vi "robot_dis.vi"() -> ()   [LabVIEW 2014]
uses:
  <vilib>/robotics/Controls/2D Rangefinder/NI_Robotics_2D Rangefinder.xctl
  <vilib>/Utility/error.llb/DialogType.ctl
  <vilib>/picture/3D Picture Control/Object/Create Object (drawable).vi
  <vilib>/picture/3D Picture Control/Object/Add Object (reference).vi
  <vilib>/picture/3D Picture Control/NI_3D Picture Control.lvlib
panel:
  out "StartChannelRecord":bool
  out "StartChannelRecord 3":bool
  out "StartChannelRecord 2":bool
  in  "AUTO":bool
  out "三维图片":refnum<vi>(3d-picture)
  out "当前方向":u8
  in  "云台枚举":enum16{"停", "上", "下", "左", "右"}(ring)
  in  "Color 2":T1={"Red"=1.0, "Green"=0.0, "Blue"=0.0, "Alpha"=1.0} caption="颜色"
  in  "Color":T1={"Red"=1.0, "Green"=0.0, "Blue"=0.0, "Alpha"=1.0} caption="颜色"
  out "小车启动":bool
  out "Lidar_two":i32
  in  "选项卡控件":T2
  out "当前速度":u16
  out "当前拉力":u16
  out "前距离(cm)":u16(slide) scale=0.0..10000.0
  out "后距离(cm)":u16(slide) scale=0.0..10000.0
  out "PITCH":i32
  out "BANK":i32
  out "HEANDING":i32
  out "当前方向":enum16{"停", "上", "下", "左", "右"}(ring)
  in  "开始后录像":bool
  in  "开始主录像":bool
  in  "开始前录像":bool
  out "前距离警告":bool
  out "后距离警告":bool
  in  "车 上":bool
  in  "车下":bool
  in  "车左":bool
  in  "加速":bool
  in  "减速":bool
  in  "车右":bool
  in  "焦距缩进":bool
  in  "焦距拉远":bool
  in  "焦点远":bool
  in  "焦点近":bool
  in  "云台右":bool
  in  "云台上":bool
  in  "云台左":bool
  in  "云台下":bool
  in  "切换备用电池":bool
  in  "绕线盘停止":bool
  in  "绕线盘反转":bool
  in  "绕线盘正转":bool
  in  "绕线转速":u16(slide) step=1 scale=500.0..10000.0
  in  "LED4":u8(slide) step=1 scale=0.0..100.0
  in  "LED3":u8(slide) step=1 scale=0.0..100.0
  in  "LED2":u8(slide) step=1 scale=0.0..100.0
  in  "LED1":u8(slide) step=1 scale=0.0..100.0
  in  "拉力上限":u16(slide) scale=0.0..2000.0
  in  "拉力下限":u16(slide) scale=0.0..2000.0
  in  "退出绕线盘模式":bool
  out "控制器":dbl(slide) scale=10.0..13.0
  out "绕线盘":dbl(slide) scale=10.0..13.0 scale format="%.3f"
  out "布尔 3":bool=TRUE
  out "StartChannelRealPlay":bool
  in  "Lidar_data":cluster{"数组":dbl[], "数组 2":dbl[][]}
  out "Rangefinder Indicator":cluster{"angle":dbl[], "distance":dbl[][]}(xcontrol)
  out "扫描质量":u8
  out "Lidar_size":u16
  in  "distance":dbl[](array[numeric])
  in  "angle":dbl[](array[numeric])
  out "数值 2":u8 format="%x"
  out "x或y?":u8 format="%x"
  out "x = y?":bool
  out "无符号字节数组 2":u8[](array[numeric])
  out "动力":dbl(slide) scale=10.0..13.0
  in  "控制电量":dbl(slide) scale=0.0..100.0
  in  "主摄像头":refnum<k7>(container)
  in  "后摄像头":refnum<k7>(container)
  out "Login 2":i32
  out "前摄像头":bool
  out "后摄像头":bool
  out "Login":i32
  in  "前摄像头":refnum<k7>(container)
  in  "缩放":dbl(knob)=2.2771854734286614 scale=0.0..10.0
  in  "方向枚举":enum16{"停", "上", "下", "左", "右"}(ring)
  out "和":u8
  out "小车锁定":u8
  out "数据传输":bool
  in  "数据输入":string
  in  "QUIT":bool
  in  "WRITE":bool
  # "TETRAELC--机器人测试平台V0.1"
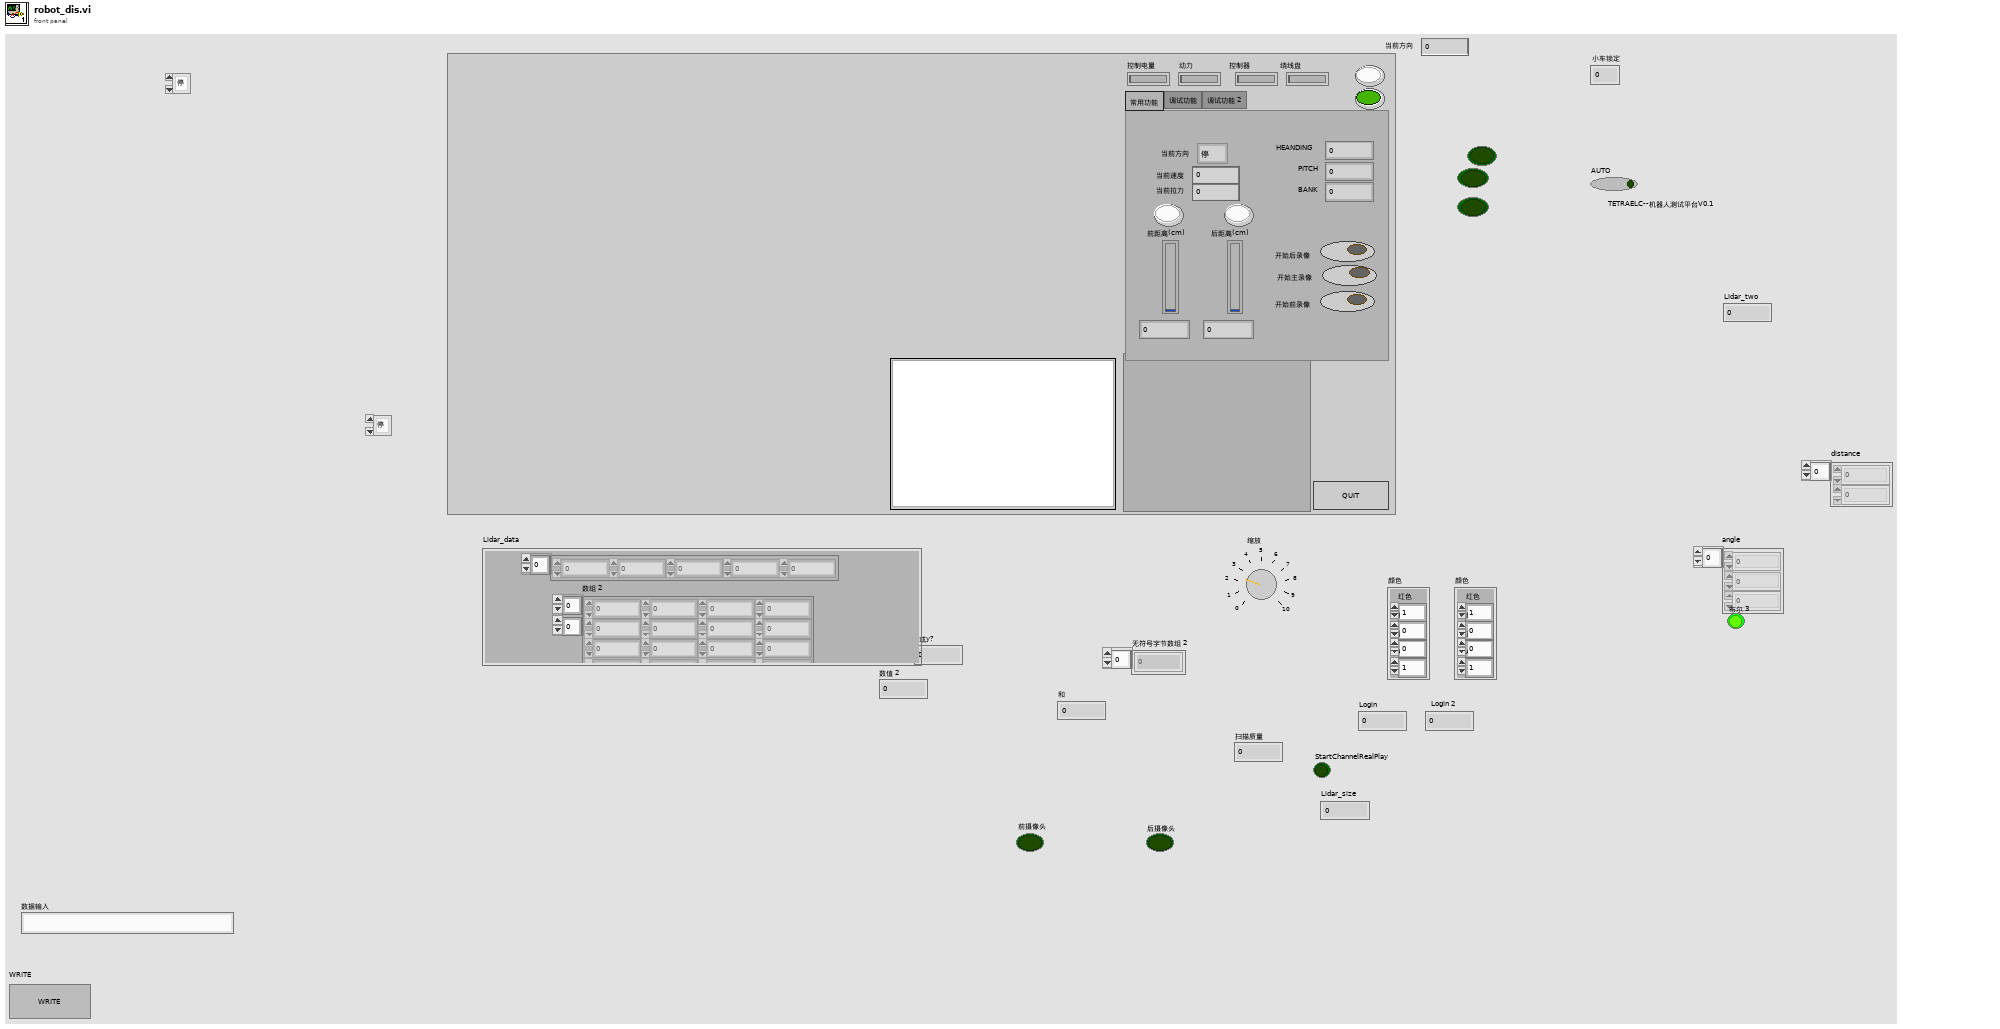
[diagram p1: front panel]
types:
  T1 = cluster{"Red":sgl, "Green":sgl, "Blue":sgl, "Alpha":sgl}
  T2 = typedef "选项卡.ctl" = enum32{"常用功能", "调试功能", "调试功能 2"}
  T3 = typedef "DialogType.ctl" = u16
  T4 = cluster{"Car_lock":u8, "当前方向":u8, "当前速度\n":u16, "当前拉力":u16}
  T5 = cluster{"PITCH":i32, "BANK":i32, "HEANDING":i32, "X":i32, "Y":i32, "Z":i32}
  T6 = cluster{"quality":u8, "angle":u16, "distance\n":u16}
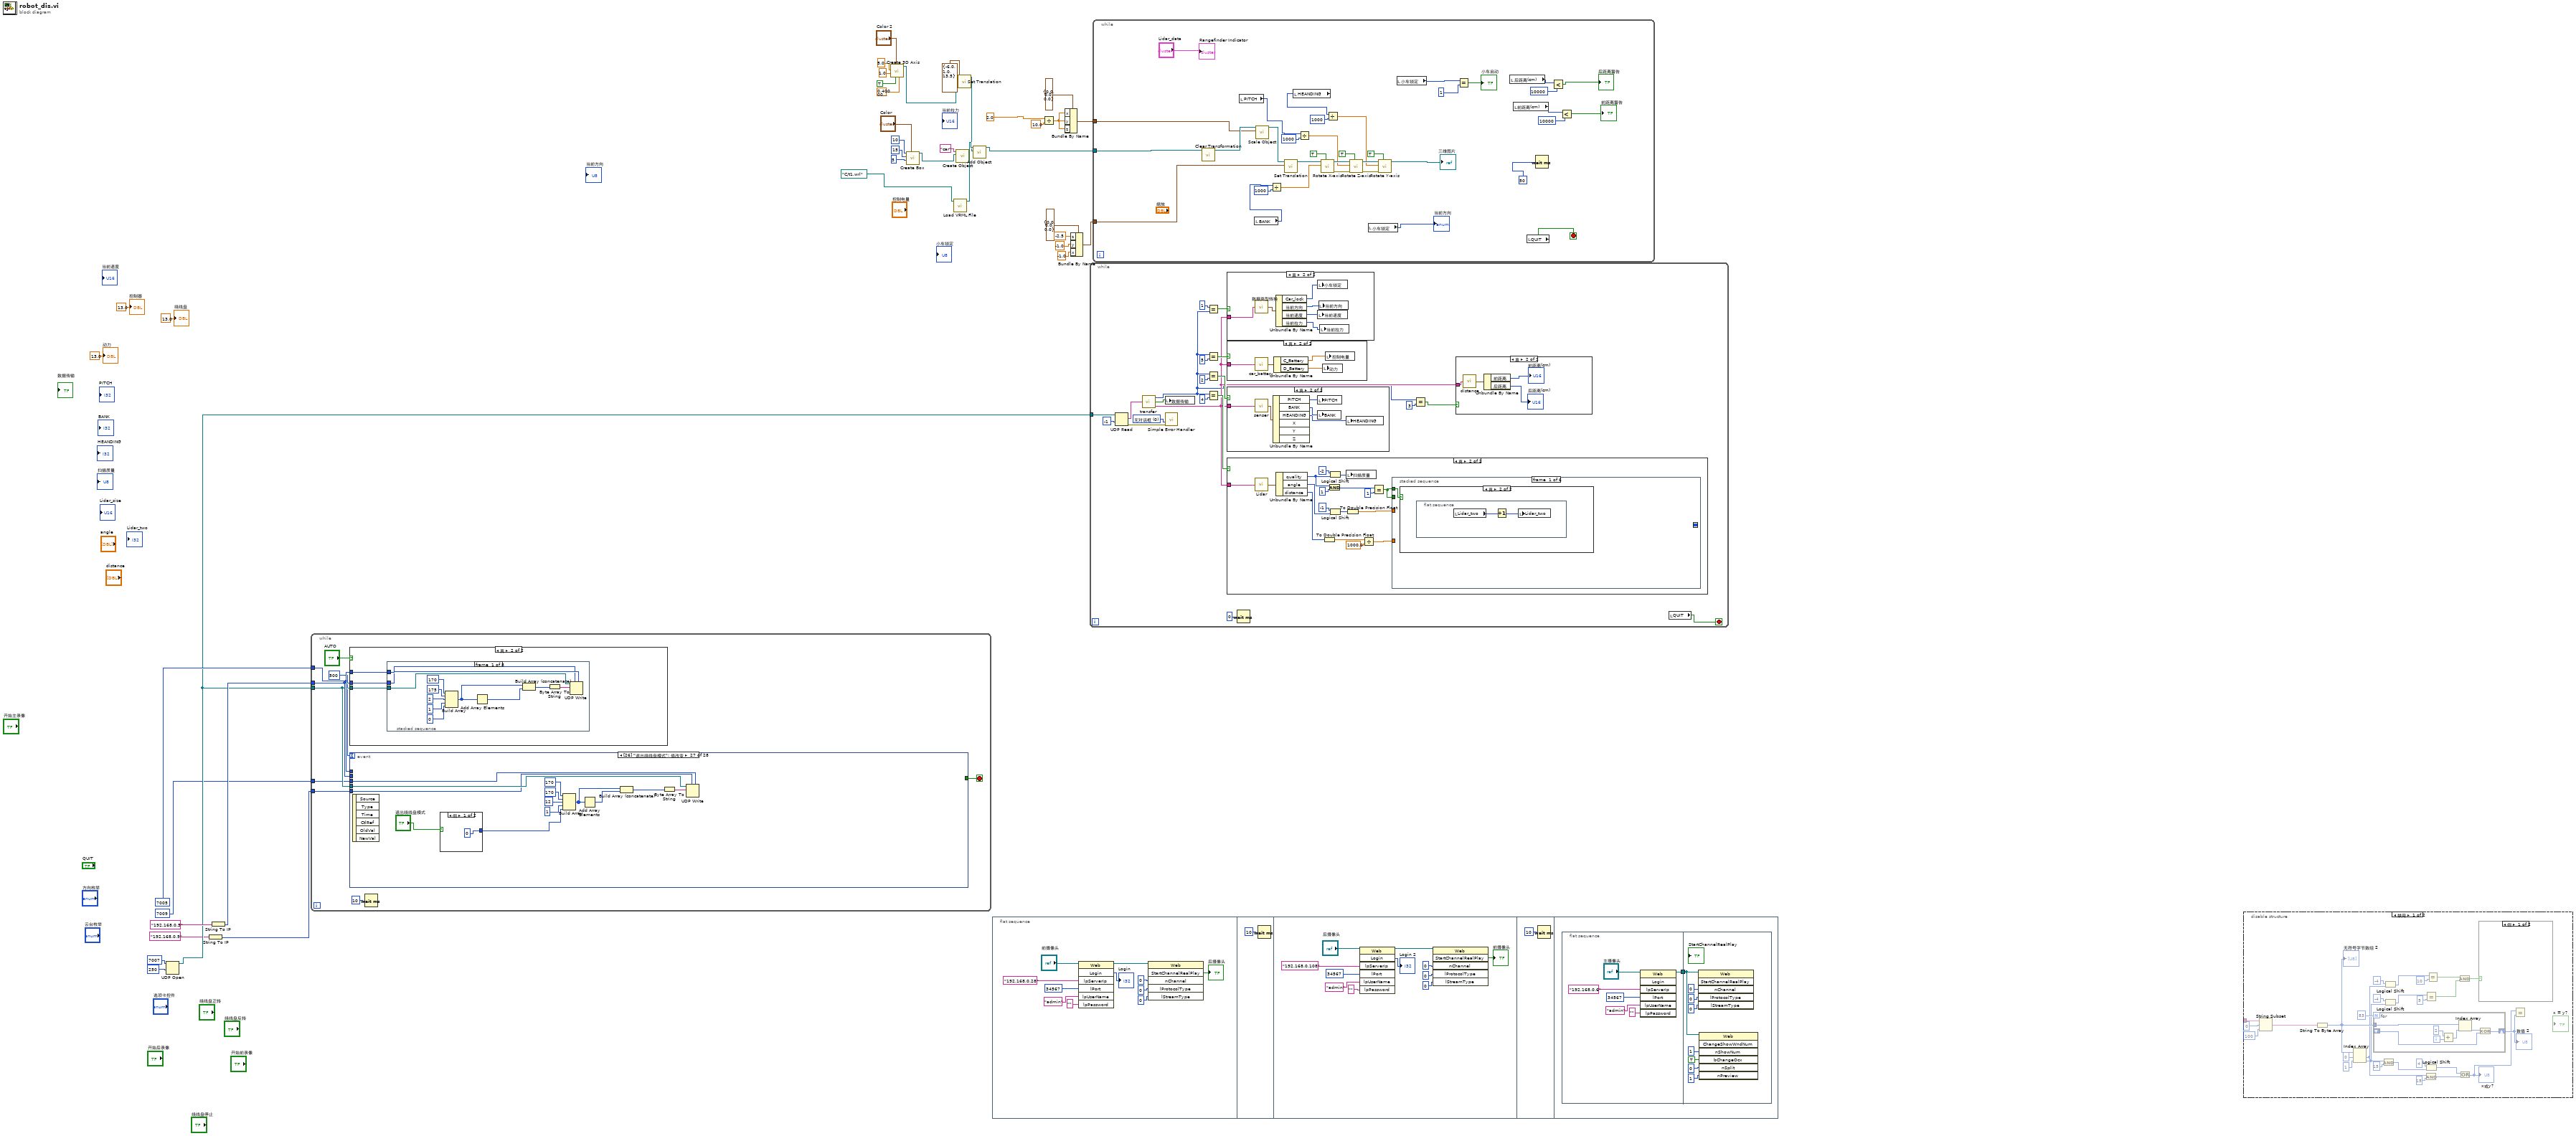
[diagram p0: block diagram]
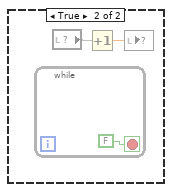
[diagram p2: hidden frame]
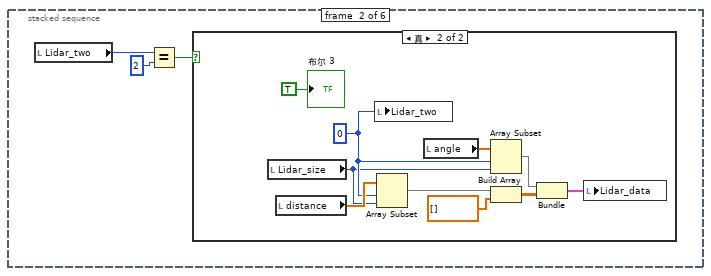
[diagram p7: hidden frame]
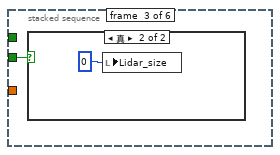
[diagram p9: hidden frame]
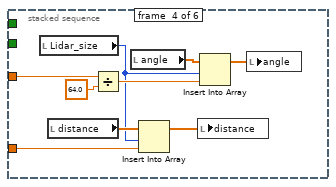
[diagram p11: hidden frame]
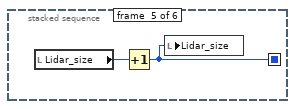
[diagram p12: hidden frame]
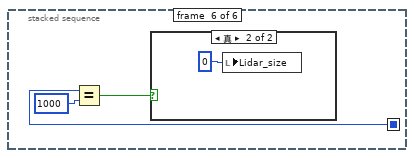
[diagram p13: hidden frame]
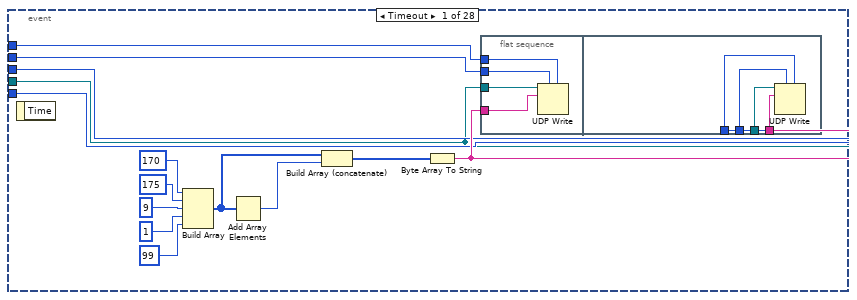
[diagram p18: hidden frame]
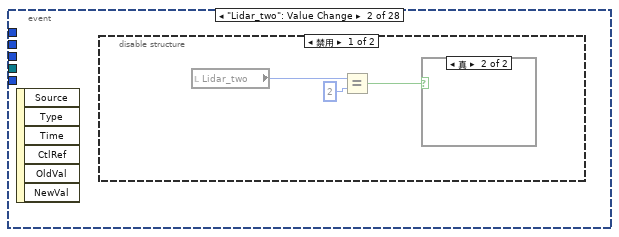
[diagram p19: hidden frame]
diagram:
  n1 = UDP Open(9:250 ("超时毫秒(25000)"), 11:u16 7007 ("本地端口")) -> (port=w26:refnum<k16>)  [unwired: 3 in, 2 out]
  n2 = String To IP(1:"192.168.0.9" ("目标主机")) -> (0:w22:u32)
  n3 = String To IP(1:"192.168.0.5" ("目标主机")) -> (0:w37:u32)
  n4 = while {
    tunnel: w26 -> [w46]
    tunnel: w37 -> [w47]
    tunnel: u16 7005 ("目标端口") -> [w48]
    tunnel: w22 -> [w41]
    tunnel: u16 7009 ("目标端口") -> [w40]
    stop <- w42 stop-if-true
    n5 = case shown="真" "AUTO" {
      tunnel: w48 -> [_ w474]
      tunnel: w47 -> [_ w473]
      tunnel: w46 -> [_ w472]
      frame False {
      }
      frame True {
        n6 = stacked-sequence {
          tunnel: w474 -> [w477 _ w488 _ w502 _ w515 _]
          tunnel: w473 -> [w476 _ w489 _ w503 _ w516 _]
          tunnel: w472 -> [w475 _ w490 _ w504 _ w514 _]
          frame #0 {
            n7 = Build Array(u8 170 ("元素"), u8 175 ("元素"), u8 2 ("元素"), u8 1 ("元素"), u8 0 ("元素")) -> (w481:u8[])
            n8 = Add Array Elements(numeric array=w481) -> (sum=w480:u8)
            n9 = Build Array (concatenate)(w481, w480) -> (w479:u8[])
            n10 = Byte Array To String(unsigned byte array=w479) -> (string=w486:string)
            n11 = UDP Write(address=w476, port or service name=w477, connection ID=w475, data in=w486) -> ()  [unwired: 2 in, 2 out]
          }
          frame #1 {
            n12 = Wait (ms)(milliseconds to wait=u32 3000 ("等待时间（毫秒）")) -> ()  [unwired: 1 out]
          }
          frame #2 {
            n13 = Build Array(u8 170 ("元素"), u8 175 ("元素"), u8 2 ("元素"), u8 1 ("元素"), u8 8 ("元素")) -> (w494:u8[])
            n14 = Add Array Elements(numeric array=w494) -> (sum=w493:u8)
            n15 = Build Array (concatenate)(w494, w493) -> (w492:u8[])
            n16 = Byte Array To String(unsigned byte array=w492) -> (string=w499:string)
            n17 = UDP Write(address=w489, port or service name=w488, connection ID=w490, data in=w499) -> ()  [unwired: 2 in, 2 out]
          }
          frame #3 {
            n18 = Wait (ms)(milliseconds to wait=u32 1000 ("等待时间（毫秒）")) -> ()  [unwired: 1 out]
          }
          frame #4 {
            n19 = Build Array(u8 170 ("元素"), u8 175 ("元素"), u8 2 ("元素"), u8 1 ("元素"), u8 1 ("元素")) -> (w508:u8[])
            n20 = Add Array Elements(numeric array=w508) -> (sum=w507:u8)
            n21 = Build Array (concatenate)(w508, w507) -> (w506:u8[])
            n22 = Byte Array To String(unsigned byte array=w506) -> (string=w512:string)
            n23 = UDP Write(address=w503, port or service name=w502, connection ID=w504, data in=w512) -> ()  [unwired: 2 in, 2 out]
          }
          frame #5 {
            n24 = Wait (ms)(milliseconds to wait=u32 3000 ("等待时间（毫秒）")) -> ()  [unwired: 1 out]
          }
          frame #6 {
            n25 = Build Array(u8 170 ("元素"), u8 175 ("元素"), u8 2 ("元素"), u8 1 ("元素"), u8 8 ("元素")) -> (w520:u8[])
            n26 = Add Array Elements(numeric array=w520) -> (sum=w519:u8)
            n27 = Build Array (concatenate)(w520, w519) -> (w518:u8[])
            n28 = Byte Array To String(unsigned byte array=w518) -> (string=w525:string)
            n29 = UDP Write(address=w516, port or service name=w515, connection ID=w514, data in=w525) -> ()  [unwired: 2 in, 2 out]
          }
          frame #7 {
            n30 = Wait (ms)(milliseconds to wait=u32 1000 ("等待时间（毫秒）")) -> ()  [unwired: 1 out]
          }
        }
      }
    }
    n31 = event shown="[26] \"退出绕线盘模式\": 值改变" {
      selector: _ -> [_ _ _ _ _ _ _ _ _ _ _ _ _ _ _ _ _ _ _ _ _ _ _ _ _ _ _ _]
      dyn-events: _ -> [_ _ _ _ _ _ _ _ _ _ _ _ _ _ _ _ _ _ _ _ _ _ _ _ _ _ _ _]
      timeout: 500 -> [_ _ _ _ _ _ _ _ _ _ _ _ _ _ _ _ _ _ _ _ _ _ _ _ _ _ _ _]
      tunnel: w46 -> [w49 _ _ _ _ w114 w131 _ _ _ _ w191 w205 w226 w250 w270 w300 w309 w331 w353 w377 w389 w399 w416 w428 w430 w440 w455]
      tunnel: w47 -> [w54 _ _ _ _ w115 w132 _ _ _ _ w192 w206 w227 w249 w271 _ w310 w332 w354 _ _ _ _ w427 _ _ w453]
      tunnel: w48 -> [w55 _ _ _ _ w116 w133 _ _ _ _ w193 w207 w228 w248 w272 _ w311 w333 w355 _ _ _ _ w426 _ _ w454]
      tunnel: [_ _ _ _ _ _ _ _ _ _ _ _ _ _ _ _ _ _ _ _ _ _ _ _ _ w429 _ _] -> w42
      tunnel: w41 -> [w51 _ _ _ _ _ _ _ _ _ _ _ _ _ _ _ w298 _ _ _ w376 w388 w401 w411 _ _ w439 _]
      tunnel: w40 -> [w50 _ _ _ _ _ _ _ _ _ _ _ _ _ _ _ w299 _ _ _ w375 w387 w400 w412 _ _ w441 _]
      event Timeout {
        n32 = event-data() -> ()  [unwired: 1 in, 1 out]
        n33 = Build Array(u8 170 ("元素"), u8 175 ("元素"), u8 9 ("元素"), u8 1 ("元素"), u8 99 ("元素")) -> (w58:u8[])
        n34 = Add Array Elements(numeric array=w58) -> (sum=w57:u8)
        n35 = Build Array (concatenate)(w58, w57) -> (w56:u8[])
        n36 = Byte Array To String(unsigned byte array=w56) -> (string=w52:string)
        n37 = flat-sequence {
          tunnel: w55 -> [w66]
          tunnel: w54 -> [w65]
          tunnel: w52 -> [w64]
          tunnel: w49 -> [w63]
          tunnel: w52 -> [w70]
          tunnel: w51 -> [w69]
          tunnel: w50 -> [w68]
          tunnel: w49 -> [w67]
          frame #0 {
            n38 = UDP Write(address=w65, port or service name=w66, connection ID=w63, data in=w64) -> ()  [unwired: 2 in, 2 out]
          }
          frame #1 {
            n39 = UDP Write(address=w69, port or service name=w68, connection ID=w67, data in=w70) -> ()  [unwired: 2 in, 2 out]
          }
        }
      }
      event "Lidar_two": Value Change {
        n40 = event-data() -> ()  [unwired: 1 in, 6 out]
        n41 = disable-structure shown="禁用" {
          frame Disabled {
            n42 = local read "Lidar_two"() -> (w73:i32)
            n43 = Equal?(x=w73, y=2) -> (x = y?=w71:bool)
            n44 = case shown="真" w71 {
              frame False {
              }
              frame True {
              }
            }
          }
          frame Enabled {
          }
        }
      }
      event "开始主录像": Value Change {
        n45 = event-data() -> ()  [unwired: 1 in, 6 out]
        n46 = local read "开始主录像"() -> (w75:bool)
        n47 = local read "主摄像头"() -> (w76:refnum<k7>)
        n48 = case shown="真" w75 {
          tunnel: w76 -> [w79 w83]
          tunnel: [w77 w80] -> w74
          frame False {
            n49 = invoke class="Web" method="StopChannelRecord"(reference=w79, "nChannel"=0) -> ("StopChannelRecord"=w77:bool)  [unwired: 2 in, 3 out]
          }
          frame True {
            n50 = invoke class="Web" method="StartChannelRecord"(reference=w83, "nChannel"=0, "lpSaveFile"="D:\\main_record", "nType"=0) -> ("StartChannelRecord"=w80:bool)  [unwired: 2 in, 5 out]
          }
        }
        "StartChannelRecord" <- w74
      }
      event "开始前录像": Value Change {
        n51 = event-data() -> ()  [unwired: 1 in, 6 out]
        n52 = local read "开始前录像"() -> (w87:bool)
        n53 = local read "前摄像头"() -> (w85:refnum<k7>)
        n54 = case shown="真" w87 {
          tunnel: w85 -> [w91 w95]
          tunnel: [w88 w92] -> w86
          frame False {
            n55 = invoke class="Web" method="StopChannelRecord"(reference=w91, "nChannel"=0) -> ("StopChannelRecord"=w89:bool)  [unwired: 2 in, 3 out]
            n56 = Not(x=w89) -> (.not. x?=w88:bool)
          }
          frame True {
            n57 = invoke class="Web" method="StartChannelRecord"(reference=w95, "nChannel"=0, "lpSaveFile"="D:\\front_record", "nType"=0) -> ("StartChannelRecord"=w92:bool)  [unwired: 2 in, 5 out]
          }
        }
        "StartChannelRecord 2" <- w86
      }
      event "开始后录像": Value Change {
        n58 = event-data() -> ()  [unwired: 1 in, 6 out]
        n59 = local read "开始后录像"() -> (w99:bool)
        n60 = local read "后摄像头"() -> (w98:refnum<k7>)
        n61 = case shown="假" w99 {
          tunnel: w98 -> [w103 w107]
          tunnel: [w100 w104] -> w97
          frame False {
            n62 = invoke class="Web" method="StopChannelRecord"(reference=w103, "nChannel"=0) -> ("StopChannelRecord"=w101:bool)  [unwired: 2 in, 3 out]
            n63 = Not(x=w101) -> (.not. x?=w100:bool)
          }
          frame True {
            n64 = invoke class="Web" method="StartChannelRecord"(reference=w107, "nChannel"=0, "lpSaveFile"="D:\\back_record", "nType"=0) -> ("StartChannelRecord"=w104:bool)  [unwired: 2 in, 5 out]
          }
        }
        "StartChannelRecord 3" <- w97
      }
      event "LED1", "LED2", "LED3", "LED4": Value Change {
        n65 = event-data() -> ()  [unwired: 1 in, 6 out]
        n66 = Build Array(u8 170 ("元素"), u8 175 ("元素"), u8 4 ("元素"), u8 4 ("元素"), "LED1", "LED2", "LED3", "LED4") -> (w120:u8[])
        n67 = Add Array Elements(numeric array=w120) -> (sum=w119:u8)
        "和" <- w119
        n68 = Build Array (concatenate)(w120, w119) -> (w118:u8[])
        n69 = Byte Array To String(unsigned byte array=w118) -> (string=w113:string)
        n70 = UDP Write(address=w115, port or service name=w116, connection ID=w114, data in=w113, 9:250 ("超时毫秒(25000)")) -> ()  [unwired: 1 in, 2 out]
      }
      event "加速": Value Change; "减速": Mouse Up {
        n71 = event-data() -> ()  [unwired: 1 in, 4 out]
        n72 = Select(t=i16 1000 ("x"), s="加速", f=i16 -1000) -> (s? t:f=w126:i16)
        n73 = Split Number(x=w126) -> (hi(x)=w130:u8, lo(x)=w129:u8)
        n74 = Build Array(u8 170 ("元素"), u8 175 ("元素"), u8 3 ("元素"), u8 2 ("元素"), w130, w129) -> (w136:u8[])
        n75 = Add Array Elements(numeric array=w136) -> (sum=w135:u8)
        n76 = Build Array (concatenate)(w136, w135) -> (w134:u8[])
        n77 = Byte Array To String(unsigned byte array=w134) -> (string=w141:string)
        n78 = UDP Write(address=w132, port or service name=w133, connection ID=w131, data in=w141) -> ()  [unwired: 2 in, 2 out]
      }
      event "焦距缩进": Value Change {
        n79 = event-data() -> ()  [unwired: 1 in, 6 out]
        n80 = local read "主摄像头"() -> (w142:refnum<k7>)
        n81 = case shown="真" "焦距缩进" {
          tunnel: w142 -> [w144 w148]
          frame False {
            n82 = invoke class="Web" method="PTZCtrlStop"(reference=w144, "lChannel"=0, "lCtrlType"=9, "lSpeed"=1) -> ()  [unwired: 2 in, 6 out]
          }
          frame True {
            n83 = invoke class="Web" method="PTZCtrlStart"(reference=w148, "lChannle"=0, "lCtrlType"=9, "lSpeed"=1) -> ()  [unwired: 2 in, 6 out]
          }
        }
      }
      event "焦点远": Value Change {
        n84 = event-data() -> ()  [unwired: 1 in, 6 out]
        n85 = local read "主摄像头"() -> (w152:refnum<k7>)
        n86 = case shown="假" "焦点远" {
          tunnel: w152 -> [w154 w158]
          frame False {
            n87 = invoke class="Web" method="PTZCtrlStop"(reference=w154, "lChannel"=0, "lCtrlType"=10, "lSpeed"=1) -> ()  [unwired: 2 in, 6 out]
          }
          frame True {
            n88 = invoke class="Web" method="PTZCtrlStart"(reference=w158, "lChannle"=0, "lCtrlType"=10, "lSpeed"=1) -> ()  [unwired: 2 in, 6 out]
          }
        }
      }
      event "焦点近": Value Change {
        n89 = event-data() -> ()  [unwired: 1 in, 6 out]
        n90 = local read "主摄像头"() -> (w162:refnum<k7>)
        n91 = case shown="假" "焦点近" {
          tunnel: w162 -> [w164 w168]
          frame False {
            n92 = invoke class="Web" method="PTZCtrlStop"(reference=w164, "lChannel"=0, "lCtrlType"=11, "lSpeed"=1) -> ()  [unwired: 2 in, 6 out]
          }
          frame True {
            n93 = invoke class="Web" method="PTZCtrlStart"(reference=w168, "lChannle"=0, "lCtrlType"=11, "lSpeed"=1) -> ()  [unwired: 2 in, 6 out]
          }
        }
      }
      event "焦距拉远": Value Change {
        n94 = event-data() -> ()  [unwired: 1 in, 6 out]
        n95 = local read "主摄像头"() -> (w172:refnum<k7>)
        n96 = case shown="真" "焦距拉远" {
          tunnel: w172 -> [w174 w178]
          frame False {
            n97 = invoke class="Web" method="PTZCtrlStop"(reference=w174, "lChannel"=0, "lCtrlType"=8, "lSpeed"=1) -> ()  [unwired: 2 in, 6 out]
          }
          frame True {
            n98 = invoke class="Web" method="PTZCtrlStart"(reference=w178, "lChannle"=0, "lCtrlType"=8, "lSpeed"=1) -> ()  [unwired: 2 in, 6 out]
          }
        }
      }
      event "车 上": Value Change {
        n99 = event-data() -> ()  [unwired: 1 in, 6 out]
        n100 = flat-sequence {
          tunnel: [w198] -> w182
          frame #0 {
            n101 = case shown="真" "车 上" {
              frame False {
                n102 = local write "方向枚举"(enum16{"停", "上", "下", "左", "右"}."停") -> ()
              }
              frame True {
                n103 = local write "方向枚举"(enum16{"停", "上", "下", "左", "右"}."上") -> ()
              }
            }
          }
          frame #1 {
            n104 = local read "方向枚举"() -> (w197:enum16{"停", "上", "下", "左", "右"})
            n105 = case shown="\"上\", 默认" w197 {
              tunnel: [u8 0 ("元素") u8 1 ("元素") u8 2 ("元素") u8 3 ("元素") u8 8 ("元素")] -> w198
              frame "上", Default {
              }
              frame "下" {
              }
              frame "左" {
              }
              frame "右" {
              }
              frame "停" {
              }
            }
          }
        }
        n106 = Build Array(u8 170 ("元素"), u8 175 ("元素"), u8 2 ("元素"), u8 1 ("元素"), w182) -> (w185:u8[])
        n107 = Add Array Elements(numeric array=w185) -> (sum=w184:u8)
        n108 = Build Array (concatenate)(w185, w184) -> (w183:u8[])
        n109 = Byte Array To String(unsigned byte array=w183) -> (string=w190:string)
        n110 = UDP Write(address=w192, port or service name=w193, connection ID=w191, data in=w190) -> ()  [unwired: 2 in, 2 out]
      }
      event "云台上": Value Change {
        n111 = event-data() -> ()  [unwired: 1 in, 6 out]
        n112 = flat-sequence {
          tunnel: [w220] -> w204
          frame #0 {
            n113 = case shown="假" "云台上" {
              frame False {
                n114 = local write "云台枚举"(enum16{"停", "上", "下", "左", "右"}."停") -> ()
              }
              frame True {
                n115 = local write "云台枚举"(enum16{"停", "上", "下", "左", "右"}."上") -> ()
              }
            }
          }
          frame #1 {
            n116 = local read "云台枚举"() -> (w219:enum16{"停", "上", "下", "左", "右"})
            n117 = case shown="\"上\", 默认" w219 {
              tunnel: [u8 0 ("元素") u8 1 ("元素") u8 2 ("元素") u8 3 ("元素") u8 8 ("元素")] -> w220
              frame "上", Default {
              }
              frame "下" {
              }
              frame "左" {
              }
              frame "右" {
              }
              frame "停" {
              }
            }
          }
        }
        n118 = Build Array(u8 170 ("元素"), u8 175 ("元素"), u8 5 ("元素"), u8 1 ("元素"), w204) -> (w210:u8[])
        n119 = Add Array Elements(numeric array=w210) -> (sum=w209:u8)
        n120 = Build Array (concatenate)(w210, w209) -> (w208:u8[])
        n121 = Byte Array To String(unsigned byte array=w208) -> (string=w215:string)
        n122 = UDP Write(address=w206, port or service name=w207, connection ID=w205, data in=w215) -> ()  [unwired: 2 in, 2 out]
      }
      event "云台下": Value Change {
        n123 = event-data() -> ()  [unwired: 1 in, 6 out]
        n124 = flat-sequence {
          tunnel: [w242] -> w229
          frame #0 {
            n125 = case shown="假" "云台下" {
              frame False {
                n126 = local write "云台枚举"(enum16{"停", "上", "下", "左", "右"}."停") -> ()
              }
              frame True {
                n127 = local write "云台枚举"(enum16{"停", "上", "下", "左", "右"}."上") -> ()
              }
            }
          }
          frame #1 {
            n128 = local read "云台枚举"() -> (w241:enum16{"停", "上", "下", "左", "右"})
            n129 = case shown="\"下\"" w241 {
              tunnel: [u8 0 ("元素") u8 1 ("元素") u8 2 ("元素") u8 3 ("元素") u8 8 ("元素")] -> w242
              frame "上", Default {
              }
              frame "下" {
              }
              frame "左" {
              }
              frame "右" {
              }
              frame "停" {
              }
            }
          }
        }
        n130 = Build Array(u8 170 ("元素"), u8 175 ("元素"), u8 5 ("元素"), u8 1 ("元素"), w229) -> (w232:u8[])
        n131 = Add Array Elements(numeric array=w232) -> (sum=w231:u8)
        n132 = Build Array (concatenate)(w232, w231) -> (w230:u8[])
        n133 = Byte Array To String(unsigned byte array=w230) -> (string=w237:string)
        n134 = UDP Write(address=w227, port or service name=w228, connection ID=w226, data in=w237) -> ()  [unwired: 2 in, 2 out]
      }
      event "云台左": Value Change {
        n135 = event-data() -> ()  [unwired: 1 in, 6 out]
        n136 = flat-sequence {
          tunnel: [w264] -> w251
          frame #0 {
            n137 = case shown="真" "云台左" {
              frame False {
                n138 = local write "云台枚举"(enum16{"停", "上", "下", "左", "右"}."停") -> ()
              }
              frame True {
                n139 = local write "云台枚举"(enum16{"停", "上", "下", "左", "右"}."左") -> ()
              }
            }
          }
          frame #1 {
            n140 = local read "云台枚举"() -> (w263:enum16{"停", "上", "下", "左", "右"})
            n141 = case shown="\"下\"" w263 {
              tunnel: [u8 0 ("元素") u8 1 ("元素") u8 2 ("元素") u8 3 ("元素") u8 8 ("元素")] -> w264
              frame "上", Default {
              }
              frame "下" {
              }
              frame "左" {
              }
              frame "右" {
              }
              frame "停" {
              }
            }
          }
        }
        n142 = Build Array(u8 170 ("元素"), u8 175 ("元素"), u8 5 ("元素"), u8 1 ("元素"), w251) -> (w254:u8[])
        n143 = Add Array Elements(numeric array=w254) -> (sum=w253:u8)
        n144 = Build Array (concatenate)(w254, w253) -> (w252:u8[])
        n145 = Byte Array To String(unsigned byte array=w252) -> (string=w259:string)
        n146 = UDP Write(address=w249, port or service name=w248, connection ID=w250, data in=w259) -> ()  [unwired: 2 in, 2 out]
      }
      event "云台右": Value Change {
        n147 = event-data() -> ()  [unwired: 1 in, 6 out]
        n148 = flat-sequence {
          tunnel: [w286] -> w273
          frame #0 {
            n149 = case shown="假" "云台右" {
              frame False {
                n150 = local write "云台枚举"(enum16{"停", "上", "下", "左", "右"}."停") -> ()
              }
              frame True {
                n151 = local write "云台枚举"(enum16{"停", "上", "下", "左", "右"}."左") -> ()
              }
            }
          }
          frame #1 {
            n152 = local read "云台枚举"() -> (w285:enum16{"停", "上", "下", "左", "右"})
            n153 = case shown="\"下\"" w285 {
              tunnel: [u8 0 ("元素") u8 1 ("元素") u8 2 ("元素") u8 3 ("元素") u8 8 ("元素")] -> w286
              frame "上", Default {
              }
              frame "下" {
              }
              frame "左" {
              }
              frame "右" {
              }
              frame "停" {
              }
            }
          }
        }
        n154 = Build Array(u8 170 ("元素"), u8 175 ("元素"), u8 5 ("元素"), u8 1 ("元素"), w273) -> (w276:u8[])
        n155 = Add Array Elements(numeric array=w276) -> (sum=w275:u8)
        n156 = Build Array (concatenate)(w276, w275) -> (w274:u8[])
        n157 = Byte Array To String(unsigned byte array=w274) -> (string=w281:string)
        n158 = UDP Write(address=w271, port or service name=w272, connection ID=w270, data in=w281) -> ()  [unwired: 2 in, 2 out]
      }
      event "拉力上限", "拉力下限": Value Change {
        n159 = event-data() -> ()  [unwired: 1 in, 6 out]
        n160 = Split Number(x="拉力上限") -> (hi(x)=w297:u8, lo(x)=w296:u8)
        n161 = Split Number(x="拉力下限") -> (hi(x)=w293:u8, lo(x)=w292:u8)
        n162 = Build Array(u8 170 ("元素"), u8 170 ("元素"), u8 11 ("元素"), u8 4 ("元素"), w297, w296, w293, w292) -> (w303:u8[])
        n163 = Add Array Elements(numeric array=w303) -> (sum=w302:u8)
        n164 = Build Array (concatenate)(w303, w302) -> (w301:u8[])
        n165 = Byte Array To String(unsigned byte array=w301) -> (string=w308:string)
        n166 = UDP Write(address=w298, port or service name=w299, connection ID=w300, data in=w308) -> ()  [unwired: 2 in, 2 out]
      }
      event "车下": Value Change {
        n167 = event-data() -> ()  [unwired: 1 in, 6 out]
        n168 = flat-sequence {
          tunnel: [w325] -> w312
          frame #0 {
            n169 = case shown="真" "车下" {
              frame False {
                n170 = local write "方向枚举"(enum16{"停", "上", "下", "左", "右"}."停") -> ()
              }
              frame True {
                n171 = local write "方向枚举"(enum16{"停", "上", "下", "左", "右"}."下") -> ()
              }
            }
          }
          frame #1 {
            n172 = local read "方向枚举"() -> (w324:enum16{"停", "上", "下", "左", "右"})
            n173 = case shown="\"上\", 默认" w324 {
              tunnel: [u8 0 ("元素") u8 1 ("元素") u8 2 ("元素") u8 3 ("元素") u8 8 ("元素")] -> w325
              frame "上", Default {
              }
              frame "下" {
              }
              frame "左" {
              }
              frame "右" {
              }
              frame "停" {
              }
            }
          }
        }
        n174 = Build Array(u8 170 ("元素"), u8 175 ("元素"), u8 2 ("元素"), u8 1 ("元素"), w312) -> (w315:u8[])
        n175 = Add Array Elements(numeric array=w315) -> (sum=w314:u8)
        n176 = Build Array (concatenate)(w315, w314) -> (w313:u8[])
        n177 = Byte Array To String(unsigned byte array=w313) -> (string=w320:string)
        n178 = UDP Write(address=w310, port or service name=w311, connection ID=w309, data in=w320) -> ()  [unwired: 2 in, 2 out]
      }
      event "车左": Value Change {
        n179 = event-data() -> ()  [unwired: 1 in, 6 out]
        n180 = flat-sequence {
          tunnel: [w347] -> w334
          frame #0 {
            n181 = case shown="真" "车左" {
              frame False {
                n182 = local write "方向枚举"(enum16{"停", "上", "下", "左", "右"}."停") -> ()
              }
              frame True {
                n183 = local write "方向枚举"(enum16{"停", "上", "下", "左", "右"}."左") -> ()
              }
            }
          }
          frame #1 {
            n184 = local read "方向枚举"() -> (w346:enum16{"停", "上", "下", "左", "右"})
            n185 = case shown="\"上\", 默认" w346 {
              tunnel: [u8 0 ("元素") u8 1 ("元素") u8 2 ("元素") u8 3 ("元素") u8 8 ("元素")] -> w347
              frame "上", Default {
              }
              frame "下" {
              }
              frame "左" {
              }
              frame "右" {
              }
              frame "停" {
              }
            }
          }
        }
        n186 = Build Array(u8 170 ("元素"), u8 175 ("元素"), u8 2 ("元素"), u8 1 ("元素"), w334) -> (w337:u8[])
        n187 = Add Array Elements(numeric array=w337) -> (sum=w336:u8)
        n188 = Build Array (concatenate)(w337, w336) -> (w335:u8[])
        n189 = Byte Array To String(unsigned byte array=w335) -> (string=w342:string)
        n190 = UDP Write(address=w332, port or service name=w333, connection ID=w331, data in=w342) -> ()  [unwired: 2 in, 2 out]
      }
      event "车右": Value Change {
        n191 = event-data() -> ()  [unwired: 1 in, 6 out]
        n192 = flat-sequence {
          tunnel: [w369] -> w356
          frame #0 {
            n193 = case shown="真" "车右" {
              frame False {
                n194 = local write "方向枚举"(enum16{"停", "上", "下", "左", "右"}."停") -> ()
              }
              frame True {
                n195 = local write "方向枚举"(enum16{"停", "上", "下", "左", "右"}."右") -> ()
              }
            }
          }
          frame #1 {
            n196 = local read "方向枚举"() -> (w368:enum16{"停", "上", "下", "左", "右"})
            n197 = case shown="\"上\", 默认" w368 {
              tunnel: [u8 0 ("元素") u8 1 ("元素") u8 2 ("元素") u8 3 ("元素") u8 8 ("元素")] -> w369
              frame "上", Default {
              }
              frame "下" {
              }
              frame "左" {
              }
              frame "右" {
              }
              frame "停" {
              }
            }
          }
        }
        n198 = Build Array(u8 170 ("元素"), u8 175 ("元素"), u8 2 ("元素"), u8 1 ("元素"), w356) -> (w359:u8[])
        n199 = Add Array Elements(numeric array=w359) -> (sum=w358:u8)
        n200 = Build Array (concatenate)(w359, w358) -> (w357:u8[])
        n201 = Byte Array To String(unsigned byte array=w357) -> (string=w364:string)
        n202 = UDP Write(address=w354, port or service name=w355, connection ID=w353, data in=w364) -> ()  [unwired: 2 in, 2 out]
      }
      event "绕线盘正转": Value Change {
        n203 = event-data() -> ()  [unwired: 1 in, 6 out]
        n204 = Build Array(u8 170 ("元素"), u8 170 ("元素"), u8 12 ("元素"), u8 1 ("元素"), u8 1 ("元素")) -> (w381:u8[])
        n205 = Add Array Elements(numeric array=w381) -> (sum=w380:u8)
        n206 = Build Array (concatenate)(w381, w380) -> (w379:u8[])
        n207 = Byte Array To String(unsigned byte array=w379) -> (string=w386:string)
        n208 = UDP Write(address=w376, port or service name=w375, connection ID=w377, data in=w386) -> ()  [unwired: 2 in, 2 out]
      }
      event "绕线盘反转": Value Change {
        n209 = event-data() -> ()  [unwired: 1 in, 6 out]
        n210 = Build Array(u8 170 ("元素"), u8 170 ("元素"), u8 12 ("元素"), u8 1 ("元素"), u8 2 ("元素")) -> (w393:u8[])
        n211 = Add Array Elements(numeric array=w393) -> (sum=w392:u8)
        n212 = Build Array (concatenate)(w393, w392) -> (w391:u8[])
        n213 = Byte Array To String(unsigned byte array=w391) -> (string=w398:string)
        n214 = UDP Write(address=w388, port or service name=w387, connection ID=w389, data in=w398) -> ()  [unwired: 2 in, 2 out]
      }
      event "绕线盘停止": Value Change {
        n215 = event-data() -> ()  [unwired: 1 in, 6 out]
        n216 = Build Array(u8 170 ("元素"), u8 170 ("元素"), u8 12 ("元素"), u8 1 ("元素"), u8 0 ("元素")) -> (w405:u8[])
        n217 = Add Array Elements(numeric array=w405) -> (sum=w404:u8)
        n218 = Build Array (concatenate)(w405, w404) -> (w403:u8[])
        n219 = Byte Array To String(unsigned byte array=w403) -> (string=w410:string)
        n220 = UDP Write(address=w401, port or service name=w400, connection ID=w399, data in=w410) -> ()  [unwired: 2 in, 2 out]
      }
      event "绕线转速": Value Change {
        n221 = event-data() -> ()  [unwired: 1 in, 6 out]
        n222 = Split Number(x="绕线转速") -> (hi(x)=w414:u8, lo(x)=w413:u8)
        n223 = Build Array(u8 170 ("元素"), u8 170 ("元素"), u8 13 ("元素"), u8 2 ("元素"), w414, w413) -> (w419:u8[])
        n224 = Add Array Elements(numeric array=w419) -> (sum=w418:u8)
        n225 = Build Array (concatenate)(w419, w418) -> (w417:u8[])
        n226 = Byte Array To String(unsigned byte array=w417) -> (string=w424:string)
        n227 = UDP Write(address=w411, port or service name=w412, connection ID=w416, data in=w424) -> ()  [unwired: 2 in, 2 out]
      }
      event "WRITE": Value Change {
        n228 = event-data() -> ()  [unwired: 1 in, 1 out]
        n229 = UDP Write(address=w427, port or service name=w426, connection ID=w428, data in="数据输入") -> ()  [unwired: 2 in, 2 out]
      }
      event "QUIT": Value Change {
        n230 = event-data() -> ()  [unwired: 1 in, 1 out]
        n231 = flat-sequence {
          tunnel: w430 -> [w434]
          tunnel: [TRUE] -> w429
          frame #0 {
            n232 = UDP Close(connection ID=w434) -> ()  [unwired: 1 in, 2 out]
            n233 = local read "前摄像头"() -> (w433:refnum<k7>)
            n234 = local read "后摄像头"() -> (w432:refnum<k7>)
            n235 = local read "主摄像头"() -> (w431:refnum<k7>)
            n236 = invoke class="Web" method="StopRealPlayAll"(reference=w433) -> ()  [unwired: 2 in, 3 out]
            n237 = invoke class="Web" method="StopRealPlayAll"(reference=w431) -> ()  [unwired: 2 in, 3 out]
            n238 = invoke class="Web" method="StopRealPlayAll"(reference=w432) -> ()  [unwired: 2 in, 3 out]
          }
          frame #1 {
            n239 = Quit LabVIEW(quit? (T)=TRUE ("退出？(T)")) -> ()
          }
        }
      }
      event "退出绕线盘模式": Value Change {
        n240 = event-data() -> ()  [unwired: 1 in, 6 out]
        n241 = case shown="假" "退出绕线盘模式" {
          tunnel: [u8 0 ("元素") u8 4 ("元素")] -> w437
          frame False {
          }
          frame True {
          }
        }
        n242 = Build Array(u8 170 ("元素"), u8 170 ("元素"), u8 12 ("元素"), u8 1 ("元素"), w437) -> (w444:u8[])
        n243 = Add Array Elements(numeric array=w444) -> (sum=w443:u8)
        n244 = Build Array (concatenate)(w444, w443) -> (w442:u8[])
        n245 = Byte Array To String(unsigned byte array=w442) -> (string=w449:string)
        n246 = UDP Write(address=w439, port or service name=w441, connection ID=w440, data in=w449) -> ()  [unwired: 2 in, 2 out]
      }
      event "切换备用电池": Value Change {
        n247 = event-data() -> ()  [unwired: 1 in, 6 out]
        n248 = flat-sequence {
          tunnel: [w457] -> w452
          tunnel: w455 -> [w463]
          tunnel: w454 -> [w462]
          tunnel: w453 -> [w461]
          tunnel: w452 -> [w460]
          frame #0 {
            n249 = case shown="假" "切换备用电池" {
              tunnel: [0 1] -> w457
              frame False {
              }
              frame True {
              }
            }
          }
          frame #1 {
            n250 = Build Array(u8 170 ("元素"), u8 175 ("元素"), u8 6 ("元素"), u8 1 ("元素"), w460) -> (w469:i32[])
            n251 = Add Array Elements(numeric array=w469) -> (sum=w470:i32)
            n252 = Build Array (concatenate)(w469, w470) -> (w471:i32[])
            n253 = Byte Array To String(unsigned byte array=w471) -> (string=w464:string)
            n254 = UDP Write(address=w461, port or service name=w462, connection ID=w463, data in=w464) -> ()  [unwired: 2 in, 2 out]
          }
        }
      }
    }
    n255 = Wait (ms)(milliseconds to wait=u32 10 ("等待时间（毫秒）")) -> ()  [unwired: 1 out]
  }
  n256 = call <vilib>:"Create 3D Axis.vi"("Character Size"=sgl 0.4, "Axis label?"=TRUE, "Color"="Color 2", "Radius"=sgl 1.0, "Length"=sgl 5.0) -> ("New Object Refnum"=w16:refnum<vi>)  [unwired: 5 in, 1 out]
  n257 = call <vilib>:"Create Box.vi"("Color"="Color", "Length Z"=5, "Length Y"=15, "Length X"=10) -> ("New Box Refnum"=w25:refnum<vi>)  [unwired: 6 in, 1 out]
  n258 = call <vilib>:"Load VRML File.vi"("Path"=path "C:/t1.wrl" ("路径")) -> ("Scene:Read Scene File"=w18:refnum<vi>)  [unwired: 9 in, 1 out]
  n259 = call-poly <vilib>:"Create Object.vi"("Geometry"=w25, "Name"="car") -> ()  [unwired: 8 in, 2 out]
  n260 = call <vilib>:"Set Translation.vi"("Translation"=cluster{"X":sgl, "Y":sgl, "Z":sgl} {"X"=-6.0, "Y"=1.0, "Z"=13.5}, "Scene Object"=w16) -> ("Translated Object"=w15:refnum<vi>)  [unwired: 8 in, 1 out]
  n261 = call-poly <vilib>:"Add Object.vi"("New Object In"=w15, "Scene Object In"=w18) -> ("Scene Object Out"=w24:refnum<vi>)  [unwired: 7 in, 2 out]
  n262 = flat-sequence {
    frame #0 {
      n263 = invoke class="Web" method="Login"(reference="前摄像头", "lpServerIp"="192.168.0.28", "lPort"=34567, "lpUserName"="admin", "lpPassword"="") -> (reference out=w531:refnum<k7>, "Login"=→"Login":i32)  [unwired: 2 in, 5 out]
      n264 = invoke class="Web" method="StartChannelRealPlay"(reference=w531, "nChannel"=0, "lProtocolType"=0, "lStreamType"=0) -> ("StartChannelRealPlay"=→"后摄像头":bool)  [unwired: 2 in, 5 out]
    }
    frame #1 {
      n265 = Wait (ms)(milliseconds to wait=u32 10 ("等待时间（毫秒）")) -> ()  [unwired: 1 out]
    }
    frame #2 {
      n266 = invoke class="Web" method="Login"(reference="后摄像头", "lpServerIp"="192.168.0.108", "lPort"=34567, "lpUserName"="admin", "lpPassword"="") -> (reference out=w545:refnum<k7>, "Login"=→"Login 2":i32)  [unwired: 2 in, 5 out]
      n267 = invoke class="Web" method="StartChannelRealPlay"(reference=w545, "nChannel"=0, "lProtocolType"=0, "lStreamType"=0) -> ("StartChannelRealPlay"=→"前摄像头":bool)  [unwired: 2 in, 5 out]
    }
    frame #3 {
      n268 = Wait (ms)(milliseconds to wait=u32 10 ("等待时间（毫秒）")) -> ()  [unwired: 1 out]
    }
    frame #4 {
      n269 = flat-sequence {
        tunnel: [w553] -> w551
        tunnel: w551 -> [w558]
        frame #0 {
          n270 = invoke class="Web" method="Login"(reference="主摄像头", "lpServerIp"="192.168.0.6", "lPort"=34567, "lpUserName"="admin", "lpPassword"="") -> (reference out=w553:refnum<k7>)  [unwired: 2 in, 6 out]
        }
        frame #1 {
          n271 = invoke class="Web" method="StartChannelRealPlay"(reference=w558, "nChannel"=0, "lProtocolType"=0, "lStreamType"=0) -> ()  [unwired: 2 in, 6 out]
          n272 = invoke class="Web" method="ChangeShowWndNum"(reference=w558, "nShowNum"=1, "bChangeOcx"=TRUE, "nSplit"=0, "nPreview"=1) -> ()  [unwired: 2 in, 7 out]
        }
      }
    }
  }
  n273 = Divide(x=2.0, y=10.0) -> (x/y=w8:dbl)
  n274 = Bundle By Name(cluster=cluster{"x":dbl, "y":dbl, "z":dbl} {"x"=0.0, "y"=0.0, "z"=0.0}, "x"=w8, "y"=w8, "z"=w8) -> (w6:cluster{"x":dbl, "y":dbl, "z":dbl})
  n275 = Bundle By Name(cluster=cluster{"x":dbl, "y":dbl, "z":dbl} {"x"=0.0, "y"=0.0, "z"=0.0}, "z"=-2.5, "y"=-1.0, "x"=-1.0) -> (w13:cluster{"x":dbl, "y":dbl, "z":dbl})
  n276 = while {
    tunnel: w26 -> [w573]
    stop <- w570 stop-if-true
    w576 = T3 0 items=["无对话框", "确定信息", "继续或停止信息", "确定信息＋警告", "继续/停止+警告"] ("type of dialog (OK msg:1)")
    n277 = UDP Read(connection ID=w573, timeout ms (25000)=-1 ("超时毫秒(25000)")) -> (data out=w577:string, error out=w575:errorcluster)  [unwired: 2 in, 3 out]
    n278 = call "transfer.vi"("输入"=w577) -> ("数值"=w567:u8, "布尔"=w572:bool, "输出"=w569:string)
    n279 = local write "数据传输"(w572) -> ()
    n280 = call <vilib>:"Simple Error Handler.vi"("type of dialog (OK msg:1)"=w576, "error in (no error)"=w575) -> ()  [unwired: 3 in, 5 out]
    n281 = Equal?(x=u8 1, y=w567) -> (x = y?=w579:bool)
    n282 = Equal?(x=w567, y=u8 5 ("x")) -> (x = y?=w583:bool)
    n283 = Equal?(x=w567, y=u8 2 ("x")) -> (x = y?=w581:bool)
    n284 = Equal?(x=w567, y=u8 4 ("x")) -> (x = y?=w585:bool)
    n285 = case shown="真" w579 {
      tunnel: w569 -> [_ w650]
      frame False {
      }
      frame True {
        n286 = call "数据类型转换.vi"("read buffer"=w650) -> ("输出簇"=w649:T4)
        n287 = Unbundle By Name(w649) -> ("Car_lock"=w648:u8, "当前方向"=w647:u8, "当前速度"=w646:u16, "当前拉力"=w645:u16)
        n288 = local write "小车锁定"(w648) -> ()
        n289 = local write "当前速度"(w646) -> ()
        n290 = local write "当前方向"(w647) -> ()
        n291 = local write "当前拉力"(w645) -> ()
      }
    }
    n292 = case shown="真" w583 {
      tunnel: w569 -> [_ w654]
      frame False {
      }
      frame True {
        n293 = call "car_battery.vi"("read buffer"=w654) -> ("输出簇"=w653:cluster{"C_Battery":dbl, "D_Battery\n":dbl})
        n294 = Unbundle By Name(w653) -> ("C_Battery"=w652:dbl, "D_Battery"=w651:dbl)
        n295 = local write "动力"(w651) -> ()
        n296 = local write "控制电量"(w652) -> ()
      }
    }
    n297 = case shown="真" w581 {
      tunnel: w569 -> [_ w644]
      frame False {
      }
      frame True {
        n298 = call "senser.vi"("read buffer"=w644) -> ("输出簇"=w643:T5)
        n299 = Unbundle By Name(w643) -> ("PITCH"=w642:i32, "BANK"=w641:i32, "HEANDING"=w640:i32)  [unwired: 3 out]
        n300 = local write "PITCH"(w642) -> ()
        n301 = local write "BANK"(w641) -> ()
        n302 = local write "HEANDING"(w640) -> ()
      }
    }
    n303 = case shown="真" w585 {
      tunnel: w569 -> [_ w606]
      frame False {
      }
      frame True {
        n304 = call "Lidar.vi"("read buffer"=w606) -> ("输出簇"=w605:T6)
        n305 = Unbundle By Name(w605) -> ("quality"=w597:u8, "angle"=w601:u16, "distance"=w593:u16)
        n306 = To Double Precision Float(number=w593) -> (double precision float=w592:dbl)
        n307 = And(x=w597, y=u8 1) -> (x .and. y?=w596:u8)
        n308 = Logical Shift(y=i16 -2, x=w597) -> (x << y=w602:u8)
        n309 = Logical Shift(y=i16 -1, x=w601) -> (x << y=w600:u16)
        n310 = local write "扫描质量"(w602) -> ()
        n311 = To Double Precision Float(number=w600) -> (double precision float=w598:dbl)
        n312 = Divide(x=w592, y=1000.0) -> (x/y=w590:dbl)
        n313 = Equal?(x=w596, y=u8 1) -> (x = y?=w594:bool)
        n314 = stacked-sequence {
          seq-local: [_ _ _ _ w634 _] -> [_ _ _ _ _ w637]
          tunnel: w594 -> [w607 _ _ _ _ _]
          tunnel: w594 -> [_ _ w623 _ _ _]
          tunnel: w598 -> [_ _ _ w630 _ _]
          tunnel: w590 -> [_ _ _ w625 _ _]
          frame #0 {
            n315 = case shown="真" w607 {
              frame False {
              }
              frame True {
                n316 = flat-sequence {
                  frame #0 {
                    n317 = local read "Lidar_two"() -> (w609:i32)
                    n318 = Increment(x=w609) -> (x+1=w608:i32)
                    n319 = local write "Lidar_two"(w608) -> ()
                  }
                }
              }
            }
          }
          frame #1 {
            n320 = local read "Lidar_two"() -> (w612:i32)
            n321 = Equal?(x=w612, y=2) -> (x = y?=w610:bool)
            n322 = case shown="真" w610 {
              frame False {
              }
              frame True {
                w620 = 0 ("Lidar_two")
                n323 = local read "Lidar_size"() -> (w619:u16)
                n324 = local read "distance"() -> (w621:dbl[])
                n325 = local write "Lidar_two"(w620) -> ()
                n326 = Array Subset(array=w621, index=w620, length=w619) -> (w618:dbl[])
                n327 = local read "angle"() -> (w622:dbl[])
                n328 = Array Subset(array=w622, index=w620, length=w619) -> (w616:dbl[])
                n329 = Build Array(w618, dbl[] [] ("元素")) -> (w615:dbl[][])
                n330 = Bundle(w616, w615) -> (w613:cluster{dbl[], dbl[][]})  [unwired: 1 in]
                n331 = local write "Lidar_data"(w613) -> ()
                "布尔 3" <- TRUE
              }
            }
          }
          frame #2 {
            n332 = case shown="真" w623 {
              frame False {
              }
              frame True {
                n333 = local write "Lidar_size"(u8 0 ("Lidar_size")) -> ()
              }
            }
          }
          frame #3 {
            n334 = local read "Lidar_size"() -> (w626:u16)
            n335 = local read "distance"() -> (w627:dbl[])
            n336 = Divide(x=w630, y=64.0) -> (x/y=w629:dbl)
            n337 = local read "angle"() -> (w633:dbl[])
            n338 = Insert Into Array(array=w627, index=w626, new element=w625) -> (w628:dbl[])
            n339 = local write "distance"(w628) -> ()
            n340 = Insert Into Array(array=w633, index=w626, new element=w629) -> (w632:dbl[])
            n341 = local write "angle"(w632) -> ()
          }
          frame #4 {
            n342 = local read "Lidar_size"() -> (w635:u16)
            n343 = Increment(x=w635) -> (x+1=w634:u16)
            n344 = local write "Lidar_size"(w634) -> ()
          }
          frame #5 {
            n345 = Equal?(x=w637, y=u16 1000) -> (x = y?=w636:bool)
            n346 = case shown="真" w636 {
              frame False {
              }
              frame True {
                n347 = local write "Lidar_size"(u16 0 ("Lidar_size")) -> ()
              }
            }
          }
        }
      }
    }
    n348 = Wait (ms)(milliseconds to wait=u32 0 ("等待时间（毫秒）")) -> ()  [unwired: 1 out]
    n349 = Equal?(x=w567, y=u8 3 ("x")) -> (x = y?=w566:bool)
    n350 = case shown="真" w566 {
      tunnel: w569 -> [_ w589]
      frame False {
      }
      frame True {
        n351 = call "distance.vi"("read buffer"=w589) -> ("输出簇"=w588:cluster{"前距离\n":u16, "后距离":u16})
        n352 = Unbundle By Name(w588) -> ("前距离"=→"前距离(cm)":u16, "后距离"=→"后距离(cm)":u16)
      }
    }
    n353 = local read "QUIT"() -> (w570:bool)
  }
  n354 = while {
    tunnel: w24 -> [w672]
    tunnel: w13 -> [w663]
    tunnel: w6 -> [w662]
    stop <- w689 stop-if-true
    n355 = call <vilib>:"Clear Transformation.vi"("Object Refnum In"=w672) -> ("Object Refnum Out"=w673:refnum<vi>)  [unwired: 9 in, 1 out]
    n356 = local read "PITCH"() -> (w666:i32)
    n357 = local read "BANK"() -> (w665:i32)
    n358 = call <vilib>:"Scale Object.vi"("Scale"=w662, "Scene.Object In"=w673) -> ("Scene.Object Out"=w688:refnum<vi>)  [unwired: 8 in, 1 out]
    n359 = Divide(x=w665, y=1000) -> (x/y=w676:dbl)
    n360 = call <vilib>:"Set Translation.vi"("Translation"=w663, "Scene Object"=w688) -> ("Translated Object"=w685:refnum<vi>)  [unwired: 8 in, 1 out]
    n361 = local read "HEANDING"() -> (w664:i32)
    n362 = Divide(x=w666, y=1000) -> (x/y=w677:dbl)
    n363 = call <vilib>:"Rotate X-axis.vi"("Relative?"=TRUE, "angle"=w676, "Scene Object In"=w685) -> ("error out"=w684:errorcluster, "Scene Object Out"=w683:refnum<vi>)  [unwired: 7 in]
    n364 = Divide(x=w664, y=1000) -> (x/y=w675:dbl)
    n365 = call <vilib>:"Rotate Z-axis.vi"("Relative?"=TRUE, "error in (no error)"=w684, "angle"=w677, "Scene Object In"=w683) -> ("error out"=w680:errorcluster, "Scene Object Out"=w679:refnum<vi>)  [unwired: 6 in]
    n366 = local read "小车锁定"() -> (→"当前方向":u8)
    n367 = call <vilib>:"Rotate Y-axis.vi"("Relative?"=TRUE, "error in (no error)"=w680, "angle"=w675, "Scene Object In"=w679) -> ("Scene Object Out"=→"三维图片":refnum<vi>)  [unwired: 6 in, 1 out]
    n368 = local read "小车锁定"() -> (w670:u8)
    n369 = Equal?(x=w670, y=u8 1) -> (x = y?=→"小车启动":bool)
    n370 = local read "后距离(cm)"() -> (w660:u16)
    n371 = local read "前距离(cm)"() -> (w656:u16)
    n372 = local read "QUIT"() -> (w689:bool)
    n373 = Wait (ms)(milliseconds to wait=u32 50 ("等待时间（毫秒）")) -> ()  [unwired: 1 out]
    n374 = Less?(x=w660, y=u16 10000) -> (x < y?=→"后距离警告":bool)
    n375 = Less?(x=w656, y=u16 10000) -> (x < y?=→"前距离警告":bool)
    "Rangefinder Indicator" <- "Lidar_data"
  }
  n376 = disable-structure shown="禁用" {
    disable-tunnel: _ -> [w707 _]
    frame Disabled {
      n377 = String Subset(string=w707, offset (0)=0 ("长度（剩余）"), length (rest)=100 ("长度（剩余）")) -> (substring=w717:string)
      n378 = String To Byte Array(string=w717) -> (unsigned byte array=w704:u8[])
      "无符号字节数组 2" <- w704
      n379 = Index Array(array=w704, index #1=0 ("索引"), index #2=1 ("索引")) -> (element #1=w695:u8, element #2=w694:u8)
      n380 = for {
        N: 83 -> [_]
        tunnel: w704 -> [w724]
        shift-right: [w719] -> w693
        shift-left: _ -> [w718]
        i -> [w723]
        n381 = Add(x=2, y=w723) -> (x+y=w721:i32)
        n382 = Index Array(array=w724, index=w721) -> (element=w720:u8)
        n383 = Exclusive Or(1:w718, 2:w720) -> (0:w719:u8)
      }
      "数值 2" <- w693
      n384 = And(x=w694, y=u8 15) -> (x .and. y?=w697:u8)
      n385 = Logical Shift(y=i16 -4, x=w695) -> (x << y=w710:u8)
      n386 = Logical Shift(y=i16 -4, x=w694) -> (x << y=w708:u8)
      n387 = Equal?(x=w708, y=u8 5) -> (x = y?=w705:bool)
      n388 = Logical Shift(y=i16 4, x=w697) -> (x << y=w699:u8)
      n389 = And(x=w695, y=u8 15) -> (x .and. y?=w698:u8)
      n390 = Equal?(x=w710, y=u8 10) -> (x = y?=w706:bool)
      n391 = And(x=w706, y=w705) -> (x .and. y?=w691:bool)
      n392 = Or(x=w699, y=w698) -> (x .or. y?=w692:u8)
      "x或y?" <- w692
      n393 = case shown="假" w691 {
        frame False {
        }
        frame True {
          n394 = while {
            stop <- FALSE stop-if-true
          }
          n395 = local read item#-1() -> (w726)
          n396 = Increment(x=w726) -> (x+1=w725:dbl)
          n397 = local write item#-1(w725) -> ()
        }
      }
      n398 = Equal?(x=w692, y=w693) -> ()  [unwired: 1 out]
    }
    frame Enabled {
    }
  }
  "动力" <- 13.0 ("动力")
  "绕线盘" <- 13.0 ("绕线盘")
  "控制器" <- 13.0 ("控制器")
